vi "etc_XCITE_SwitchXCite.vi"(8 "error in (no error)":errorcluster {"code" format="%x"}, 9 "bOn":bool, 10 "bUseCommonOnOff":bool, 11 "h":u64) -> (0 "error out":errorcluster {"code" format="%x"}, 2 "ErrorMessage":i32 format="%x", 3 "h out":u64)   [LabVIEW 2019, in "XCite.lvlib"]
doc: "Switch Xcite on or off using common switch or individual channel."
uses:
  XCite.lvlib
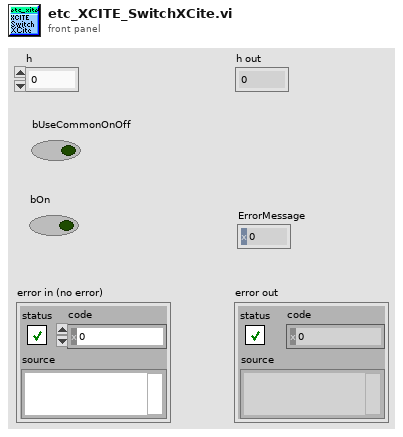
[diagram p1: front panel]
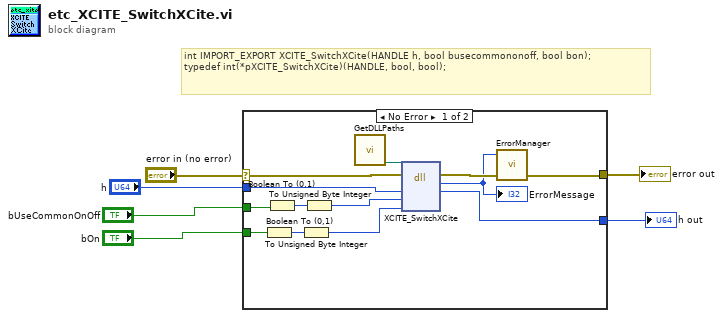
[diagram p0: block diagram]
diagram:
  # "int IMPORT_EXPORT XCITE_SwitchXCite(HANDLE h, bool busecommononoff, bool bon);\ntypedef int(*pXCITE_SwitchXCite)(HANDLE, bool, bool);"
  n1 = case shown="No Error" "error in (no error)" {
    selector: "error in (no error)" -> [w19 w21]
    tunnel: [w17 w21] -> w6
    tunnel: "h" -> [w15 w20]
    tunnel: [w14 w20] -> w4
    tunnel: "bUseCommonOnOff" -> [w10 _]
    tunnel: "bOn" -> [w9 _]
    frame No Error {
      n2 = Boolean To (0,1)(Boolean=w9) -> (0, 1=w8:i16)
      n3 = Boolean To (0,1)(Boolean=w10) -> (0, 1=w12:i16)
      n4 = To Unsigned Byte Integer(number=w8) -> (unsigned 8bit integer=w7:u8)
      n5 = To Unsigned Byte Integer(number=w12) -> (unsigned 8bit integer=w11:u8)
      n6 = call "GetDLLPaths.vi"() -> ("etc_xcite_path"=w13:path)  [unwired: 8 in, 3 out]
      n7 = dll-call lib="C:/LabVIEWDevFall2024/pco.labview/labview_sdk/runtime/bin64/etc_xcite.dll" fn="XCITE_SwitchXCite"(path in=w13, error in=w19, "h"=w15, "bUseCommonOnOff"=w11, "bOn"=w7) -> (error out=w18:errorcluster, "return type"=w16:i32, "h"=w14:u64)  [unwired: 3 in, 1 out]
      "ErrorMessage" <- w16
      n8 = call "ErrorManager.vi"("error in (no error)"=w18, "error code"=w16) -> ("error out"=w17:errorcluster)  [unwired: 2 in, 1 out]
    }
    frame Error {
    }
  }
  "error out" <- w6
  "h out" <- w4
